vi "check_if_array_of_empty_strings.vi"(11 "array":string[](array[string])) -> (3 "Not empty?":bool)   [LabVIEW 2019]
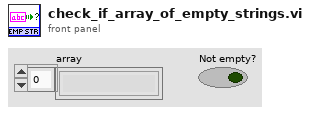
[diagram p1: front panel]
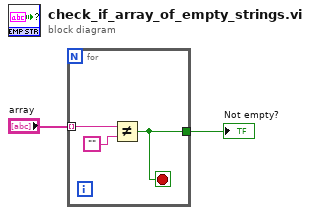
[diagram p0: block diagram]
diagram:
  n1 = for {
    tunnel: "array" -> [w5] mode=indexing
    tunnel: [w4] -> w1
    stop <- w4 stop-if-true
    n2 = Not Equal?(x=w5, y="") -> (x != y?=w4:bool)
  }
  "Not empty?" <- w1
